vi "Interpolate 2D Scattered_Nearest.vi"(0 "X":dbl[](array[numeric]), 5 "Y":dbl[](array[numeric]), 7 "Z":dbl[](array[numeric]), 9 "Xi":dbl[](array[numeric]), 11 "Yi":dbl[](array[numeric])) -> (4 "Zi":dbl[](array[numeric]), 15 "error":i32)   [LabVIEW 2020, in "NI_AAL_Interpolation.lvlib"]
uses:
  <vilib>/gmath/NI_AAL_Interpolation.lvlib
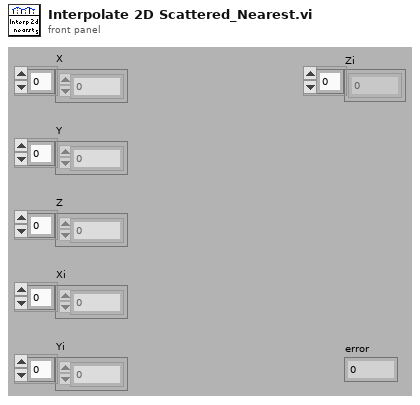
[diagram p1: front panel]
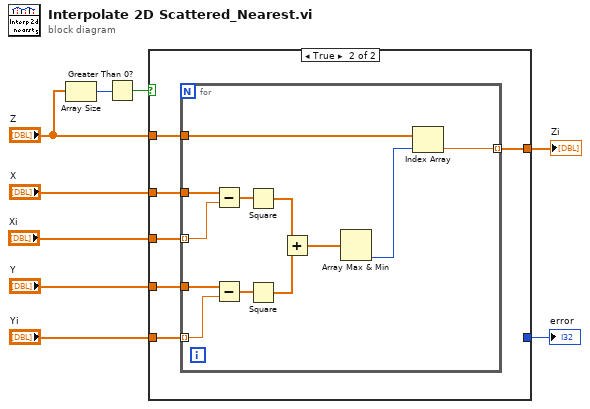
[diagram p0: block diagram]
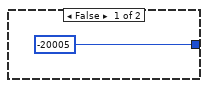
[diagram p2: hidden frame]
diagram:
  n1 = Array Size(array="Z") -> (size(s)=w3:i32)
  n2 = Greater Than 0?(x=w3) -> (x > 0?=w2:bool)
  n3 = case shown="True" w2 {
    tunnel: "Xi" -> [_ w16]
    tunnel: "Yi" -> [_ w15]
    tunnel: "X" -> [_ w14]
    tunnel: "Y" -> [_ w13]
    tunnel: [_ w12] -> w5
    tunnel: "Z" -> [_ w11]
    tunnel: [-20005 _] -> w1
    frame False {
    }
    frame True {
      n4 = for {
        tunnel: w16 -> [w27] mode=indexing
        tunnel: w15 -> [w25] mode=indexing
        tunnel: w14 -> [w28]
        tunnel: w13 -> [w26]
        tunnel: w11 -> [w19]
        tunnel: [w17] -> w12 mode=indexing
        n5 = Subtract(x=w28, y=w27) -> (x-y=w24:dbl[])
        n6 = Subtract(x=w26, y=w25) -> (x-y=w23:dbl[])
        n7 = Square(x=w24) -> (x^2=w22:dbl[])
        n8 = Square(x=w23) -> (x^2=w21:dbl[])
        n9 = Add(x=w22, y=w21) -> (x+y=w20:dbl[])
        n10 = Array Max & Min(array=w20) -> (min index (indices)=w18:i32)  [unwired: 3 out]
        n11 = Index Array(array=w19, index=w18) -> (element=w17:dbl)
      }
    }
  }
  "Zi" <- w5
  "error" <- w1
